vi "ScanZeemanWith1762WithPumpingHWT2.vi"() -> ()   [LabVIEW 2012]
uses:
  <vilib>/Instr/_visa.llb/VISA Configure Serial Port (Instr).vi
  <vilib>/Utility/file.llb/Write To Spreadsheet File (DBL).vi
panel:
  in  "RF pulse length (Units 1us)":dbl=50.0
  in  "1762 Frequency (MHz)":dbl=82.29
  out "digital waveform out 3":digitalwaveform(waveform)={"t0"=timestamp(0 s since 1904-01-01), "dt"=1e-07, "Y"={"transitions"=[0, 2100, 2200, 2300, 2301, 2321, 2421], "data"=[[1, 1, 1, 0, 0], [1, 0, 1, 0, 0], [1, 0, 0, 0, 0], [0, 0, 0, 0, 0], [0, 0, 0, 0, 1], [0, 0, 0, 0, 0], [0, 1, 1, 0, 0]]}, "error"={"status"=FALSE, "code"=37421928, "source"=""}}
  out "10xwindow":i32
  out "10xdiscr":dbl
  out "DARK?":i32(graph)=51
  out "Counts":i32=51
  out "DARK?":bool
  out "PMT Counts":i32(graph)=3
  in  "PMT sample time":dbl=0.025
  out "Counts after 1762":i32=3
  out "OuterLoop":i32=130
  out "InnerLoop":i32=24
  in  "Frequency Step Size":dbl=100000.0
  out "Bright Events":dbl
  in  "Discriminator Level\n (Bright/Dark)":i32=12
  out "digital waveform out 2":digitalwaveform(waveform)={"t0"=timestamp(0 s since 1904-01-01), "dt"=1e-07, "Y"={"transitions"=[0, 2100, 2200, 2300, 2301, 2321, 2421], "data"=[[1, 1, 1, 0, 0], [1, 0, 1, 0, 0], [1, 0, 0, 0, 0], [0, 0, 0, 0, 0], [0, 0, 0, 0, 1], [0, 0, 0, 0, 0], [0, 1, 1, 0, 0]]}, "error"={"status"=FALSE, "code"=37421928, "source"=""}}
  in  "1762 pulse length (units of 1 us)":dbl=20.0
  in  "Comment":string="*@* DPAOM = 98MHz, B-current = 2.91Amps, Comp Coil = 3.00 Amps, Axial Voltage = 500 Volts, RF frequency = 18.105, RF power = -11dBm"
  in  "B Field":dbl=2.91
  in  "Power":dbl
  in  "Rerun BG Every\nnth freq point":dbl=20.0
  in  "PMT sample time":dbl=0.025
  out "Counts finding bright ion":dbl=51.0
  in  "BG Cutoff Limit":dbl=38.0
  in  "Runs per data point":dbl=100.0
  in  "Low Freq":dbl(slide)=2000000.0 min=500000.0 max=20000000.0 step=1000.0 scale=50000.0..20000000.0 scale format="%#.5f"
  in  "High Freq":dbl(slide)=15000000.0 min=500000.0 max=20000000.0 step=1000.0 scale=50000.0..20000000.0 scale format="%#.0f"
  out "Cur Freq":dbl=1900000.0 format="%#_8f"
  out "Path":path=path "c:/data/1762 Scans/2014-07-11_14-32-23_1762scanWithPumping.txt"
  out "Frequency Scan":cluster{dbl, dbl}[](graph)=[{15000000.0, 0.12}, {14900000.0, 0.16}, {14800000.0, 0.12}, {14700000.0, 0.04}, {14600000.0, 0.16}, {14500000.0, 0.08}, {14400000.0, 0.24}, {14300000.0, 0.08}, {14200000.0, 0.2}, {14100000.0, 0.12}, {14000000.0, 0.12}, {13900000.0, 0.04}, {13800000.0, 0.28}, {13700000.0, 0.12}, {13600000.0, 0.16}, {13500000.0, 0.16}, {13400000.0, 0.12}, {13300000.0, 0.08}, {13200000.0, 0.16}, {13100000.0, 0.2}, {13000000.0, 0.08}, {12900000.0, 0.04}, {12800000.0, 0.08}, {12700000.0, 0.0}, {12600000.0, 0.0}, {12500000.0, 0.08}, {12400000.0, 0.12}, {12300000.0, 0.12}, {12200000.0, 0.16}, {12100000.0, 0.04}, {12000000.0, 0.08}, {11900000.0, 0.12}, {11800000.0, 0.12}, {11700000.0, 0.28}, {11600000.0, 0.08}, {11500000.0, 0.2}, {11400000.0, 0.24}, {11300000.0, 0.2}, {11200000.0, 0.04}, {11100000.0, 0.24}, {11000000.0, 0.12}, {10900000.0, 0.0}, {10800000.0, 0.04}, {10700000.0, 0.04}, {10600000.0, 0.08}, {10500000.0, 0.2}, {10400000.0, 0.16}, {10300000.0, 0.2}, {10200000.0, 0.2}, {10100000.0, 0.12}, {10000000.0, 0.04}, {9900000.0, 0.0}, {9800000.0, 0.2}, {9700000.0, 0.08}, {9600000.0, 0.08}, {9500000.0, 0.12}, {9400000.0, 0.12}, {9300000.0, 0.12}, {9200000.0, 0.04}, {9100000.0, 0.2}, {9000000.0, 0.08}, {8900000.0, 0.08}, {8800000.0, 0.12}, {8700000.0, 0.12}, {8600000.0, 0.24}, {8500000.0, 0.0}, {8400000.0, 0.04}, {8300000.0, 0.16}, {8200000.0, 0.08}, {8100000.0, 0.04}, {8000000.0, 0.16}, {7900000.0, 0.12}, {7800000.0, 0.08}, {7700000.0, 0.12}, {7600000.0, 0.16}, {7500000.0, 0.08}, {7400000.0, 0.16}, {7300000.0, 0.08}, {7200000.0, 0.16}, {7100000.0, 0.16}, {7000000.0, 0.16}, {6900000.0, 0.08}, {6800000.0, 0.24}, {6700000.0, 0.08}, {6600000.0, 0.32}, {6500000.0, 0.08}, {6400000.0, 0.0}, {6300000.0, 0.16}, {6200000.0, 0.04}, {6100000.0, 0.04}, {6000000.0, 0.04}, {5900000.0, 0.16}, {5800000.0, 0.08}, {5700000.0, 0.04}, {5600000.0, 0.08}, {5500000.0, 0.0}, {5400000.0, 0.08}, {5300000.0, 0.04}, {5200000.0, 0.12}, {5100000.0, 0.0}, {5000000.0, 0.12}, {4900000.0, 0.04}, {4800000.0, 0.08}, {4700000.0, 0.08}, {4600000.0, 0.04}, {4500000.0, 0.12}, {4400000.0, 0.04}, {4300000.0, 0.12}, {4200000.0, 0.12}, {4100000.0, 0.16}, {4000000.0, 0.16}, {3900000.0, 0.08}, {3800000.0, 0.24}, {3700000.0, 0.2}, {3600000.0, 0.2}, {3500000.0, 0.16}, {3400000.0, 0.12}, {3300000.0, 0.04}, {3200000.0, 0.08}, {3100000.0, 0.12}, {3000000.0, 0.24}, {2900000.0, 0.2}, {2800000.0, 0.12}, {2700000.0, 0.08}, {2600000.0, 0.12}, {2500000.0, 0.16}, {2400000.0, 0.2}, {2300000.0, 0.04}, {2200000.0, 0.2}, {2100000.0, 0.08}, {2000000.0, 0.16}]
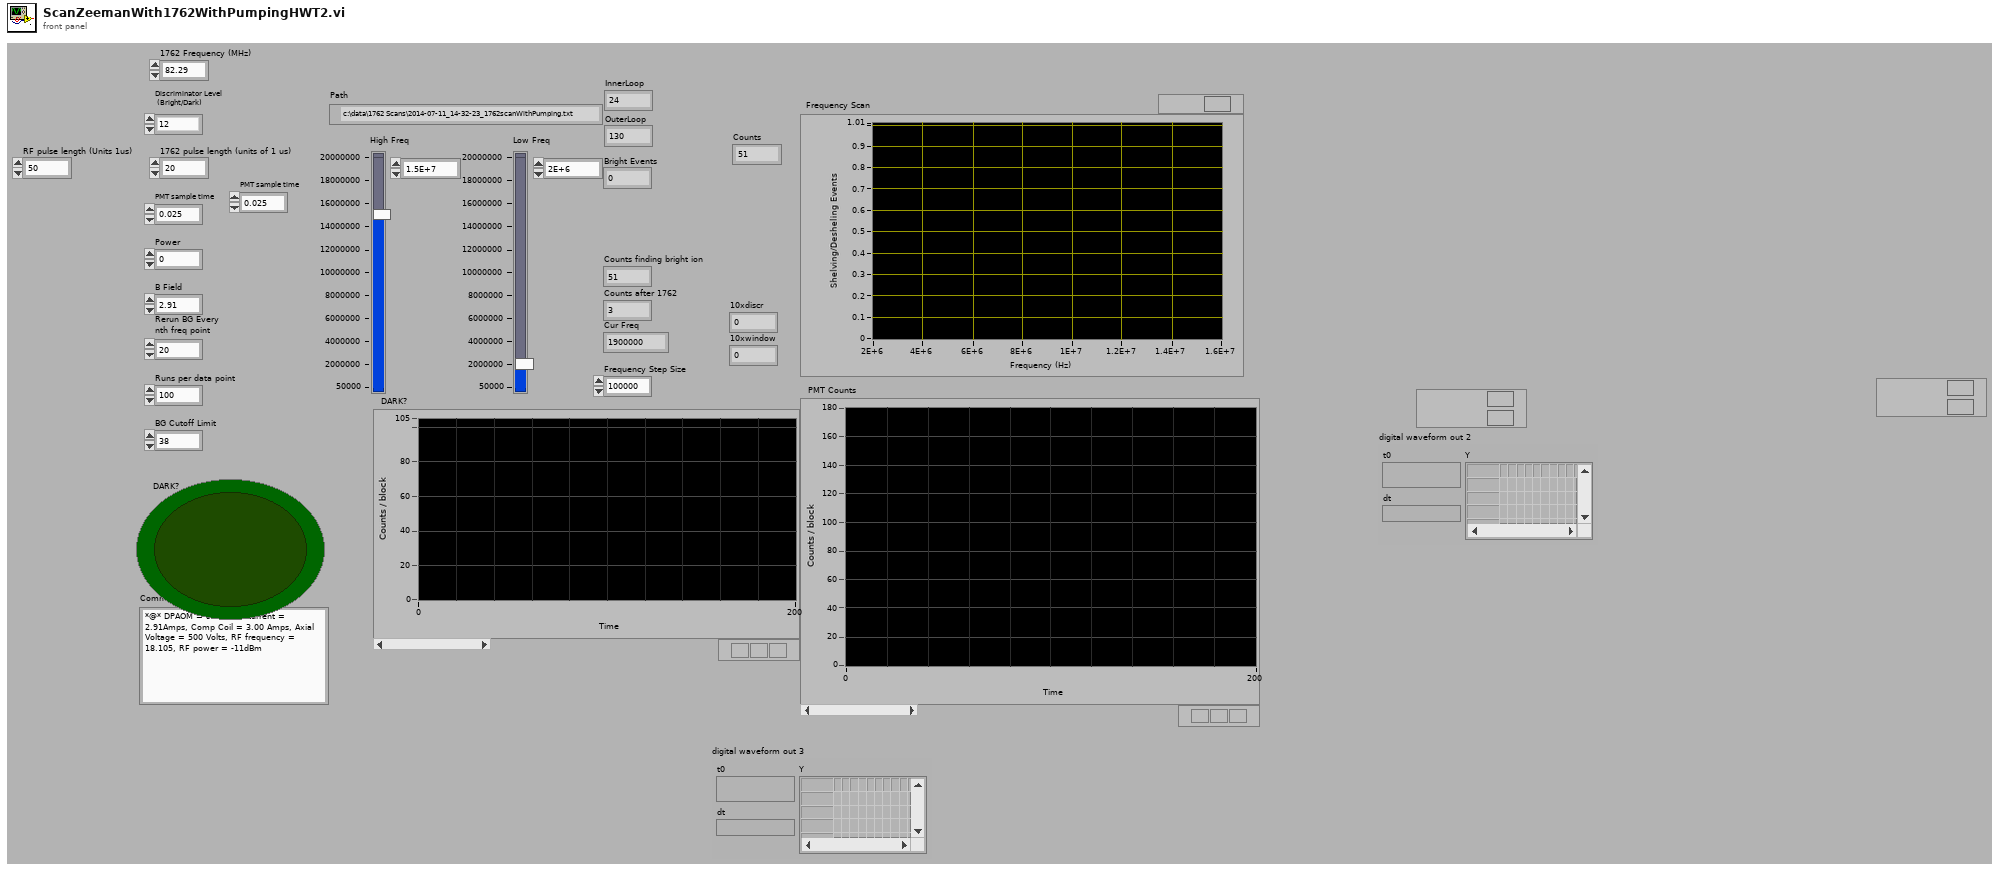
[diagram p1: front panel]
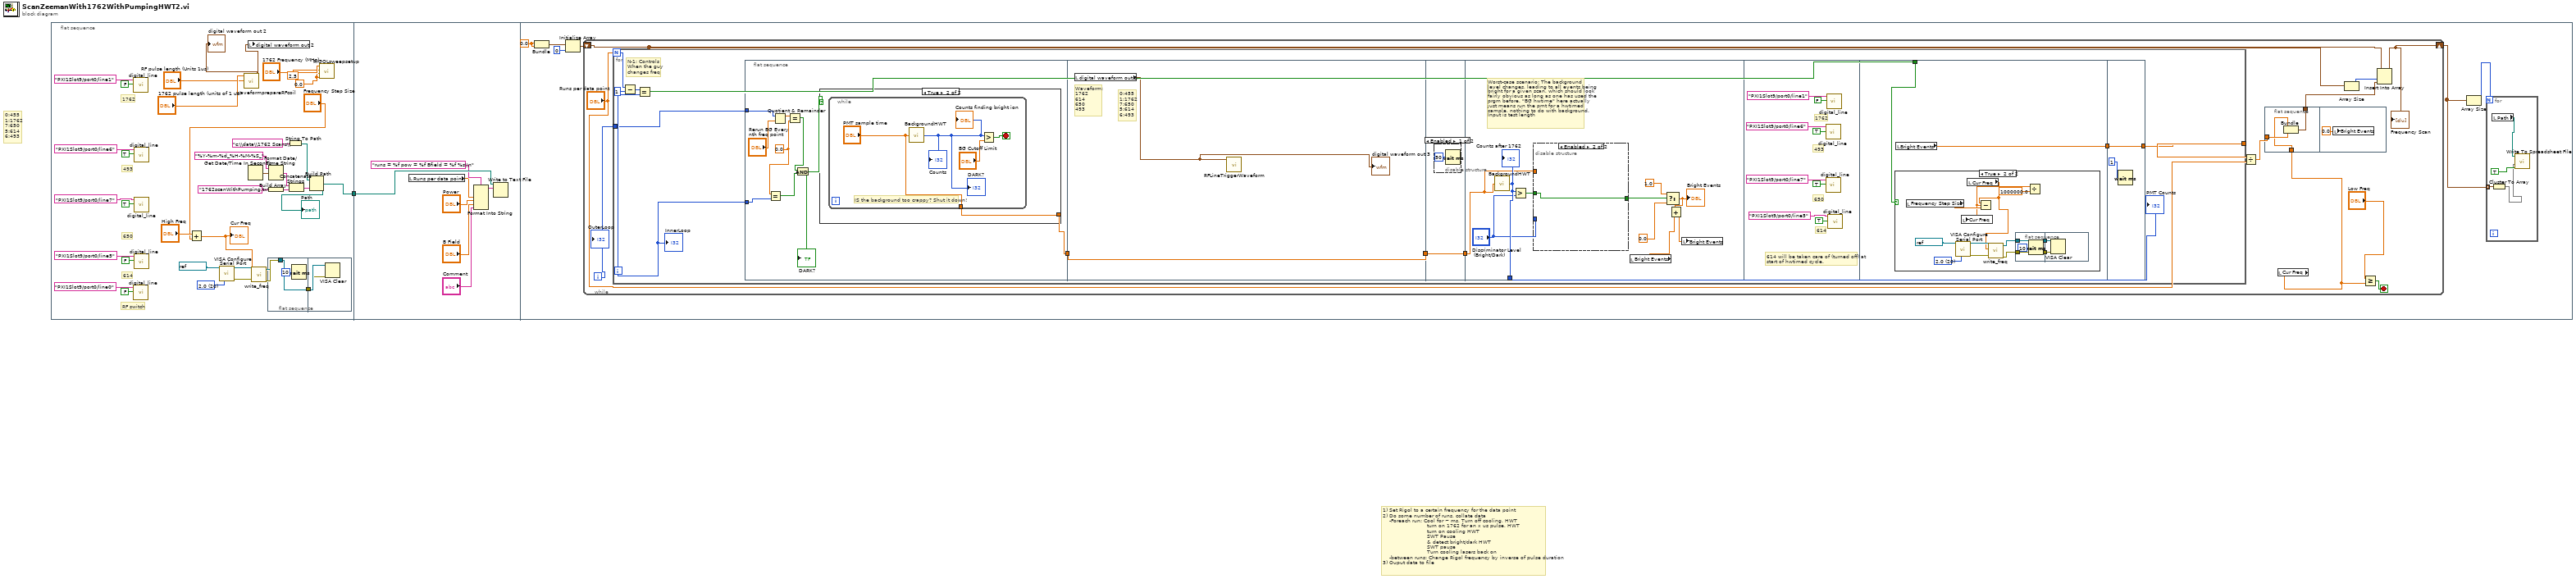
[diagram p0: block diagram]
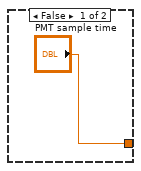
[diagram p2: hidden frame]
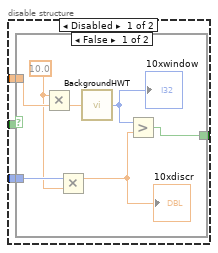
[diagram p4: hidden frame]
diagram:
  # "0:455\n1:1762\n7:650\n5:614\n6:493"
  # "1) Set Rigol to a certain frequency for the data point\n2) Do some number of runs, collate data\n    -Foreach run: Cool for ~ ms, Turn off cooling, HWT\n                           turn on 1762 for an x us pulse, HWT\n                           turn on cooling HWT\n                           SWT Pause\n                           & detect bright/dark HWT\n                           SWT pause\n                           Turn cooling lasers back on \n    -between runs: Change Rigol frequency by inverse of pulse duration\n3) Ouput data to file"
  n1 = flat-sequence {
    tunnel: [w29] -> w1
    tunnel: w1 -> [w49]
    frame #0 {
      w12 = u16 20 items=["1.0"=10, "1.5"=15, "2.0"=20] ("stop bits (10: 1 bit)")
      w16 = 0.0 ("Time (ms)")
      # "RF switch"
      # "614"
      # "650"
      # "493"
      # "1762"
      n2 = call "digital_line.vi"("Boolean"=FALSE, "lines"=tag "PXI1Slot9/port0/line1") -> ()  [unwired: 5 in, 1 out]
      n3 = call "digital_line.vi"("Boolean"=FALSE, "lines"=tag "PXI1Slot9/port0/line0") -> ()  [unwired: 5 in, 1 out]
      n4 = call "digital_line.vi"("Boolean"=TRUE, "lines"=tag "PXI1Slot9/port0/line6") -> ()  [unwired: 5 in, 1 out]
      n5 = call "digital_line.vi"("Boolean"=TRUE, "lines"=tag "PXI1Slot9/port0/line7") -> ()  [unwired: 5 in, 1 out]
      n6 = call "digital_line.vi"("Boolean"=FALSE, "lines"=tag "PXI1Slot9/port0/line5") -> ()  [unwired: 5 in, 1 out]
      n7 = Add(x="High Freq", y="Frequency Step Size") -> (x+y=w5:dbl)
      "Cur Freq" <- w5
      n8 = call-poly "VISA Configure Serial Port"("VISA resource name"=refnum<visa-resource-name> "COM1", "stop bits (10: 1 bit)"=w12) -> ("VISA resource name out"=w11:refnum<visa-resource-name>, "error out"=w10:errorcluster)  [unwired: 12 in]
      n9 = call "waveformprepareRFcoil.vi"("RF pulse length (Units 1us)"="RF pulse length (Units 1us)", "1762 pulse length (units of 1 us)"="1762 pulse length (units of 1 us)") -> ("digital waveform out 2"=w19:digitalwaveform)  [unwired: 7 in]
      "digital waveform out 2" <- w19
      n10 = local write "digital waveform out 2"(w19) -> ()
      n11 = Get Date/Time In Seconds() -> (seconds since 1Jan1904=w31:timestamp)
      n12 = call "write_freq.vi"("error in (no error)"=w10, "number"=w5, "VISA Refnum in"=w11) -> ("error out"=w9:errorcluster, "VISA Refnum out"=w8:refnum<visa-resource-name>)  [unwired: 7 in]
      n13 = flat-sequence {
        tunnel: w9 -> [w39]
        tunnel: w8 -> [w40]
        tunnel: [w40] -> w15
        tunnel: [w39] -> w14
        tunnel: w15 -> [w42]
        tunnel: w14 -> [w41]
        frame #0 {
          n14 = Wait (ms)(milliseconds to wait=u32 10) -> ()  [unwired: 1 out]
        }
        frame #1 {
          n15 = VISA Clear(VISA resource name=w42, error in (no error)=w41) -> ()  [unwired: 2 out]
        }
      }
      n16 = Format Date/Time String(time format string (%c)="%Y-%m-%d_%H-%M-%S_", seconds (now)=w31) -> (date/time string=w33:string)  [unwired: 1 in]
      n17 = Build Array("1762scanWithPumping.txt") -> (w36:string[])
      n18 = String To Path(string="c:\\data\\1762 Scans\\") -> (path=w37:path)
      n19 = Concatenate Strings(w33, w36) -> (w35:string)
      n20 = Build Path(base path=w37, name or relative path=w35) -> (appended path=w29:path)
      "Path" <- w29
      n21 = call "RIGOLsweepsetup.vi"("AP Sweep Width (MHz)"=w16, "Time (ms)"=w16, "Amplitude (Vpp)"=2.5, "Frequency (MHz)"="1762 Frequency (MHz)") -> ()  [unwired: 8 in]
    }
    frame #1 {
      n22 = local read "Runs per data point"() -> (w46:dbl)
      n23 = Format Into String(format string="runs = %f pow = %f Bfield = %f %s\\n", w46, "Power", "B Field", "Comment") -> (resulting string=w47:string)  [unwired: 2 in, 1 out]
      n24 = Write to Text File(file (use dialog)=w49, text=w47) -> ()  [unwired: 2 in, 3 out]
    }
    frame #2 {
      w54 = 0.0
      n25 = Bundle(w54, w54) -> (w55:cluster{dbl, dbl})  [unwired: 1 in]
      n26 = Initialize Array(w55, 0) -> (w52:cluster{dbl, dbl}[])
      n27 = while {
        shift-right: [w66] -> w50
        shift-left: w52 -> [w67]
        i -> [w65]
        stop <- w69 stop-if-true
        n28 = for {
          N: "Runs per data point" -> [w83]
          tunnel: [w82] -> w62
          tunnel: w65 -> [w79]
          i -> [w80]
          # "N-1: Controls\nWhen the guy\nchanges freq"
          n29 = Subtract(x=w83, y=1) -> (x-y=w86:i32)
          n30 = Equal?(x=w86, y=w80) -> (x = y?=w84:bool)
          n31 = flat-sequence {
            tunnel: w80 -> [w93]
            tunnel: w79 -> [w88]
            tunnel: [w87] -> w78
            tunnel: [w103] -> w75
            tunnel: w78 -> [w103]
            tunnel: [w104] -> w76
            tunnel: w75 -> [w104]
            tunnel: w76 -> [w108]
            tunnel: [w110] -> w77
            tunnel: w84 -> [w137]
            tunnel: [w138] -> w81
            tunnel: [w157] -> w82
            tunnel: w81 -> [w157]
            frame #0 {
              w92 = 0.0 ("x")
              n32 = Equal?(x=w92, y=w93) -> (x = y?=w90:bool)
              n33 = Quotient & Remainder(x=w88, y="Rerun BG Every\nnth freq point") -> (x-y*floor(x/y)=w94:dbl)  [unwired: 1 out]
              n34 = Equal?(x=w94, y=w92) -> (x = y?=w91:bool)
              n35 = And(x=w91, y=w90) -> (x .and. y?=w89:bool)
              "DARK?" <- w89
              n36 = case shown="True" w89 {
                tunnel: ["PMT sample time" w97] -> w87
                frame False {
                }
                frame True {
                  n37 = while {
                    tunnel: ["PMT sample time"] -> w97
                    stop <- w100 stop-if-true
                    # "IS the background too crappy? Shut it down!"
                    n38 = call "BackgroundHWT.vi"("Sample Time(seconds)"="PMT sample time") -> ("Counts"=w98:i32)
                    "Counts finding bright ion" <- w98
                    "Counts" <- w98
                    "DARK?" <- w98
                    n39 = Greater?(x=w98, y="BG Cutoff Limit") -> (0:w100:bool)
                  }
                }
              }
            }
            frame #1 {
              # "0:455\n1:1762\n7:650\n5:614\n6:493"
              # "Waveform:\n1762\n614\n650\n493"
              n40 = local read "digital waveform out 2"() -> (w102:digitalwaveform)
              "digital waveform out 3" <- w102
              n41 = call "RFLineTriggerWaveform.vi"("digital waveform in"=w102) -> ()  [unwired: 11 in]
            }
            frame #2 {
              n42 = disable-structure shown="Enabled" {
                frame Enabled {
                  n43 = Wait (ms)(milliseconds to wait=u32 50) -> ()  [unwired: 1 out]
                }
                frame Disabled {
                }
              }
            }
            frame #3 {
              # "Worst-case scenario: The background\nlevel changes, leading to all events being\nbright for a given scan, which should look\nfairly obvious as long as one has used the\nprgm before. \"BG hwtime\" here actually\njust means run the pmt for a hwtimed\nsample, nothing to do with background.\nInput is test length"
              n44 = call "BackgroundHWT.vi"("Sample Time(seconds)"=w108) -> ("Counts"=w110:i32)
              "Counts after 1762" <- w110
              n45 = Greater?(x=w110, y="Discriminator Level\n (Bright/Dark)") -> (0:w109:bool)
              n46 = disable-structure shown="Enabled" {
                disable-tunnel: w109 -> [w119 w128]
                disable-tunnel: [w118 w128] -> w106
                disable-tunnel: w108 -> [w117 _]
                disable-tunnel: "Discriminator Level\n (Bright/Dark)" -> [w116 _]
                frame Disabled {
                  n47 = case shown="False" w119 {
                    selector: w119 -> [_ w127]
                    tunnel: [w122 w127] -> w118
                    tunnel: w117 -> [w126 _]
                    tunnel: w116 -> [w123 _]
                    frame False {
                      w120 = 10.0 ("x")
                      n48 = Multiply(x=w120, y=w126) -> (x*y=w125:dbl)
                      n49 = Multiply(x=w123, y=w120) -> (x*y=w121:dbl)
                      "10xdiscr" <- w121
                      n50 = call "BackgroundHWT.vi"("Sample Time(seconds)"=w125) -> ("Counts"=w124:i32)
                      "10xwindow" <- w124
                      n51 = Greater?(x=w124, y=w121) -> (0:w122:bool)
                    }
                    frame True {
                    }
                  }
                }
                frame Enabled {
                }
              }
              n52 = local read "Bright Events"() -> (w111:dbl)
              n53 = Select(t=1.0, s=w106, f=0.0) -> (s? t:f=w113:dbl)
              "Bright Events" <- w113
              n54 = Add(x=w113, y=w111) -> (x+y=w112:dbl)
              n55 = local write "Bright Events"(w112) -> ()
            }
            frame #4 {
              # "614 will be taken care of (turned off) at\nstart of hwtimed cycle."
              # "614"
              # "650"
              # "493"
              # "1762"
              n56 = call "digital_line.vi"("Boolean"=TRUE, "lines"=tag "PXI1Slot9/port0/line6") -> ()  [unwired: 5 in, 1 out]
              n57 = call "digital_line.vi"("Boolean"=TRUE, "lines"=tag "PXI1Slot9/port0/line7") -> ()  [unwired: 5 in, 1 out]
              n58 = call "digital_line.vi"("Boolean"=FALSE, "lines"=tag "PXI1Slot9/port0/line1") -> ()  [unwired: 5 in, 1 out]
              n59 = call "digital_line.vi"("Boolean"=TRUE, "lines"=tag "PXI1Slot9/port0/line5") -> ()  [unwired: 5 in, 1 out]
            }
            frame #5 {
              n60 = case shown="True" w137 {
                frame False {
                }
                frame True {
                  w143 = u16 20 items=["1.0"=10, "1.5"=15, "2.0"=20] ("stop bits (10: 1 bit)")
                  n61 = local read "Frequency Step Size"() -> (w150:dbl)
                  n62 = call-poly "VISA Configure Serial Port"("VISA resource name"=refnum<visa-resource-name> "COM1", "stop bits (10: 1 bit)"=w143) -> ("VISA resource name out"=w144:refnum<visa-resource-name>, "error out"=w145:errorcluster)  [unwired: 12 in]
                  n63 = local read "Cur Freq"() -> (w141:dbl)
                  n64 = Subtract(x=w141, y=w150) -> (x-y=w149:dbl)
                  n65 = local write "Cur Freq"(w149) -> ()
                  n66 = call "write_freq.vi"("error in (no error)"=w145, "number"=w141, "VISA Refnum in"=w144) -> ("error out"=w146:errorcluster, "VISA Refnum out"=w147:refnum<visa-resource-name>)  [unwired: 7 in]
                  n67 = flat-sequence {
                    tunnel: w146 -> [w152]
                    tunnel: w147 -> [w153]
                    tunnel: [w153] -> w140
                    tunnel: [w152] -> w139
                    tunnel: w140 -> [w155]
                    tunnel: w139 -> [w154]
                    frame #0 {
                      n68 = Wait (ms)(milliseconds to wait=u32 10) -> ()  [unwired: 1 out]
                    }
                    frame #1 {
                      n69 = VISA Clear(VISA resource name=w155, error in (no error)=w154) -> ()  [unwired: 2 out]
                    }
                  }
                  n70 = Divide(x=w149, y=1000000.0) -> ()  [unwired: 1 out]
                }
              }
              n71 = local read "Bright Events"() -> (w138:dbl)
            }
            frame #6 {
              n72 = Wait (ms)(milliseconds to wait=u32 1) -> ()  [unwired: 1 out]
            }
          }
          "InnerLoop" <- w80
          "PMT Counts" <- w77
        }
        n73 = Divide(x=w62, y="Runs per data point") -> (x/y=w61:dbl)
        n74 = flat-sequence {
          tunnel: w61 -> [w73]
          tunnel: [w72] -> w64
          tunnel: w63 -> [w71]
          frame #0 {
            n75 = Bundle("Cur Freq"=w71, w73) -> (w72:cluster{"Cur Freq":dbl, dbl})  [unwired: 1 in]
          }
          frame #1 {
            n76 = local write "Bright Events"(0.0 ("Bright Events")) -> ()
          }
        }
        n77 = local read "Cur Freq"() -> (w63:dbl)
        n78 = Array Size(array=w67) -> (size(s)=w68:i32)
        n79 = Greater Or Equal?(x="Low Freq", y=w63) -> (x >= y?=w69:bool)
        n80 = Insert Into Array(array=w67, index=w68, new element=w64) -> (w66:cluster{dbl, dbl}[])
        "Frequency Scan" <- w66
        "OuterLoop" <- w65
      }
      n81 = Array Size(array=w50) -> (size(s)=w51:i32)
      n82 = for {
        N: w51 -> [_]
        tunnel: w50 -> [w59] mode=indexing
        n83 = local read "Path"() -> (w56:path)
        n84 = Cluster To Array(cluster=w59) -> (array=w57:dbl[])
        n85 = call-poly <vilib>:"Write To Spreadsheet File.vi"("append to file? (new file:F)"=TRUE, "1D data"=w57, "file path (dialog if empty)"=w56) -> ()  [unwired: 5 in, 1 out]
      }
    }
  }
